vi "Frequency Range to Band Number.vi"(1 "frequency range [Hz]":cluster{"low freq.":dbl, "high freq.":dbl}={"low freq."=1000.0, "high freq."=1000.0} {"high freq." min=0.001 format="%.2f"; "low freq." min=0.001 format="%.2f"}, 2 "bandwidth":T2(ring)=enum."1/3 octave", 3 "standard":T1) -> (0 "band number":cluster{"low band":i32, "high band":i32})   [LabVIEW 2017]
doc: "Converts the selected frequency range to the corresponding band number, based on the specified bandwidth and standard (ANSI or IEC).\nThe band number is based on the low and high bands specified in the frequency range cluster. A value of 0 corresponds to the reference frequency of the audio-frequency range, 1 kHz. Each successive value corresponds to the next fractional-octave band. Positive values cover the range above 1 kHz, and negative values cover the range below 1 kHz."
uses:
  <vilib>/addons/_NISVFA/_Shared subVIs/Controls/svc_Octave Standard.ctl
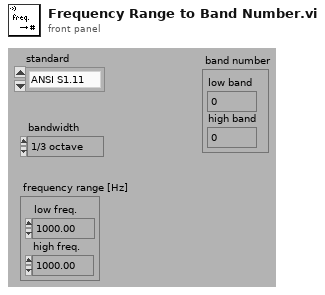
[diagram p1: front panel]
types:
  T1 = typedef "svc_Octave Standard.ctl" = enum16{"ANSI S1.11", "IEC 61260"}
  T2 = enum16{"1 octave", "1/3 octave", "1/6 octave", "1/12 octave", "1/24 octave"}
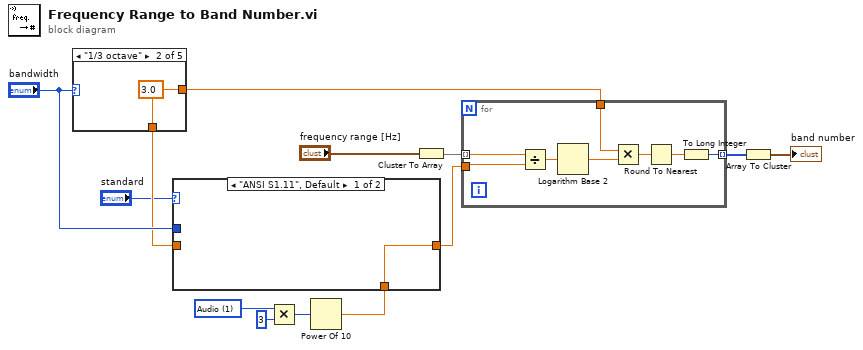
[diagram p0: block diagram]
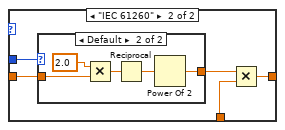
[diagram p2: hidden frame]
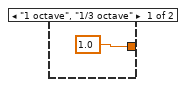
[diagram p3: hidden frame]
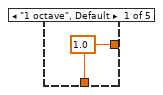
[diagram p4: hidden frame]
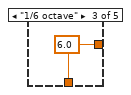
[diagram p5: hidden frame]
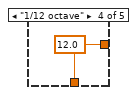
[diagram p6: hidden frame]
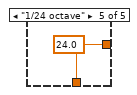
[diagram p7: hidden frame]
diagram:
  w1 = u16 1 items=["Infrasonic", "Audio", "Ultrasonic"] ("reference frequency range")
  n1 = case shown="\"1/3 octave\"" "bandwidth" {
    tunnel: [w14 w15 w16 w17 w18] -> w12
    tunnel: [w14 w15 w16 w17 w18] -> w6
    frame "1 octave", Default {
      w14 = 1.0
    }
    frame "1/3 octave" {
      w15 = 3.0
    }
    frame "1/6 octave" {
      w16 = 6.0
    }
    frame "1/12 octave" {
      w17 = 12.0
    }
    frame "1/24 octave" {
      w18 = 24.0
    }
  }
  n2 = Multiply(x=w1, y=u16 3) -> (x*y=w4:u16)
  n3 = Power Of 10(x=w4) -> (10^x=w2:dbl)
  n4 = case shown="\"ANSI S1.11\", Default" "standard" {
    tunnel: [w19 w23] -> w7
    tunnel: "bandwidth" -> [_ w24]
    tunnel: w6 -> [_ w21]
    tunnel: w2 -> [w19 w20]
    frame "ANSI S1.11", Default {
    }
    frame "IEC 61260" {
      n5 = case shown="Default" w24 {
        tunnel: [1.0 ("x") w30] -> w22
        tunnel: w21 -> [_ w27]
        frame "1 octave", "1/3 octave" {
        }
        frame Default {
          n6 = Multiply(x=2.0, y=w27) -> (x*y=w28:dbl)
          n7 = Reciprocal(x=w28) -> (1/x=w29:dbl)
          n8 = Power Of 2(x=w29) -> (2^x=w30:dbl)
        }
      }
      n9 = Multiply(x=w22, y=w20) -> (x*y=w23:dbl)
    }
  }
  n10 = Cluster To Array(cluster="frequency range [Hz]") -> (array=w10:dbl[])
  n11 = for {
    tunnel: w7 -> [w38]
    tunnel: w12 -> [w36]
    tunnel: w10 -> [w35] mode=indexing
    tunnel: [w31] -> w9 mode=indexing
    n12 = Divide(x=w35, y=w38) -> (x/y=w37:dbl)
    n13 = Logarithm Base 2(1:w37) -> (0:w34:dbl)
    n14 = Multiply(x=w36, y=w34) -> (x*y=w33:dbl)
    n15 = Round To Nearest(number=w33) -> (nearest integer value=w32:dbl)
    n16 = To Long Integer(number=w32) -> (32bit integer=w31:i32)
  }
  n17 = Array To Cluster(array=w9) -> (cluster=→"band number":cluster{"[0]":i32, "[1]":i32})
